vi "Run all tests CLI.vi"   [LabVIEW 2021]
uses:
  <vilib>/addons/_JKI Toolkits/Caraya/classes/Test Report/Test Report.lvclass
  <vilib>/addons/_JKI Toolkits/Caraya/run-tests/Run Test (Scalar Path).vi
  <vilib>/addons/_JKI Toolkits/Caraya/classes/Test Suite/Test Suite.lvclass
  <vilib>/Wiresmith Technology/G CLI/CLI Class/CLI.lvclass
  <vilib>/addons/_JKI Toolkits/Caraya/classes/Test Result/Test Result.lvclass
  <vilib>/addons/_JKI Toolkits/Caraya/Caraya.lvlib
types:
  T1 = enum32{"Invalid", "Standard", "Closed", "Hidden", "Minimized", "Maximized"}
  T2 = typedef "Caraya.lvlib/Test Result.lvclass/Node Results (Extended).ctl" = cluster{"Test Node":T3, "Assertions":T5[]}
  T3 = typedef "Caraya.lvlib/Test Result.lvclass/Test Node (Extended).ctl" = cluster{"Test Registration":T4, "Defined":bool, "Passed":bool, "properties":variant}
  T4 = typedef "Caraya.lvlib/Test Result.lvclass/Test Registration Data.ctl" = cluster{"Name":string, "Call Chain":string[], "Time Stamp":timestamp, "Test ID":string, "Caller ID":string}
  T5 = typedef "Caraya.lvlib/Test Result.lvclass/Assert Event Data (Extended).ctl" = cluster{"name":string, "passed":bool, "call-chain":string[], "test-error":errorcluster, "timestamp":timestamp, "assert-id":string, "test-id":string, "time":dbl, "message":string, "properties":variant, "measurements":variant, "user-defined":variant}
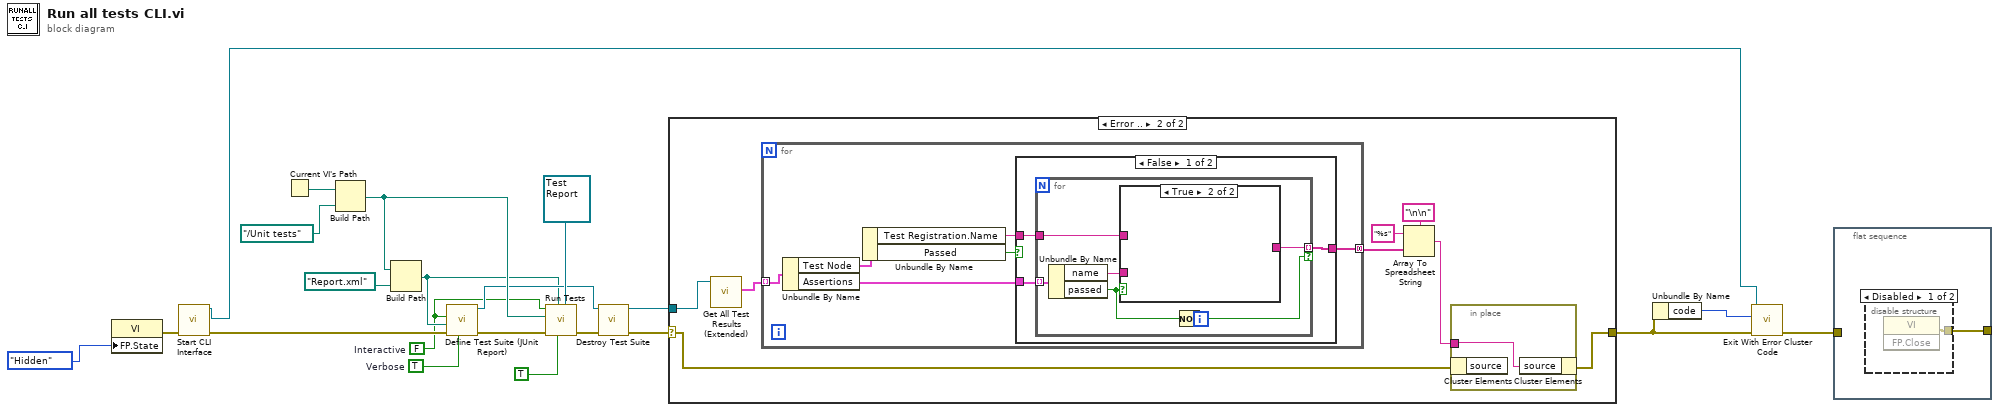
[diagram p0: block diagram]
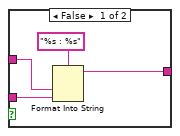
[diagram p3: hidden frame]
diagram:
  w12 = TRUE  # Verbose
  w1 = FALSE  # Interactive
  n1 = property class="VI"("FP.State"=T1."Hidden" ("Front Panel Window:State")) -> (error out=w8:errorcluster)  [unwired: 2 in, 1 out]
  n2 = call <vilib>:"Start CLI Interface.vi"("error in (no error)"=w8) -> ("error out"=w3:errorcluster, "CLI out"=w6:refnum<class "CLI.lvclass">)  [unwired: 7 in, 2 out]
  n3 = Current VI's Path() -> (path=w19:path)
  n4 = Build Path(base path=w19, name or relative path=path "../Unit tests") -> (appended path=w16:path)
  n5 = Build Path(base path=w16, name or relative path=path "Report.xml") -> (appended path=w11:path)
  n6 = call <vilib>:"Define Test Suite (JUnit Report).vi"("Verbose (F)"=w12, "error in (no error)"=w3, "Report Path"=w11, "Interactive"=w1) -> ("error out"=w10:errorcluster, "Test Suite"=w13:refnum<class "Test Suite.lvclass">)  [unwired: 5 in, 1 out]
  n7 = call-poly <vilib>:"Run Tests.vi"("Test Report"=refnum<class "Test Report.lvclass"> refnum, "Verbose"=TRUE, "Report Path"=w11, "error in"=w10, "Test Path"=w16, "Interactive (T)"=w1) -> ("error out"=w9:errorcluster)  [unwired: 4 in, 1 out]
  n8 = call-dynamic "Destroy Test Suite.vi"("error in (no error)"=w9, "Test Suite in"=w13) -> ("error out"=w5:errorcluster, "Test Suite Results"=w14:refnum<class "Test Result.lvclass">)  [unwired: 8 in]
  n9 = case shown="Error .." w5 {
    selector: w5 -> [w22 w25]
    tunnel: w14 -> [_ w30]
    tunnel: [w22 w23] -> w4
    frame No Error {
    }
    frame Error {
      n10 = call <vilib>:"Get All Test Results (Extended).vi"("Test Result in"=w30) -> ("Test Results"=w26:T2[])  [unwired: 8 in, 2 out]
      n11 = for {
        tunnel: w26 -> [w36] mode=indexing
        tunnel: [w32] -> w27 mode=concatenating
        n12 = Unbundle By Name(w36) -> ("Test Node"=w35:T3, "Assertions"=w37:T5[])
        n13 = Unbundle By Name(w35) -> ("Test Registration.Name"=w33:string, "Passed"=w34:bool)
        n14 = case shown="False" w34 {
          tunnel: w37 -> [w40 _]
          tunnel: w33 -> [w39 _]
          tunnel: [w38 _] -> w32
          frame False {
            n15 = for {
              tunnel: w40 -> [w46] mode=indexing
              tunnel: w39 -> [w44]
              tunnel: [w43] -> w38 mode=indexing if=w41
              n16 = Unbundle By Name(w46) -> ("name"=w45:string, "passed"=w42:bool)
              n17 = case shown="True" w42 {
                tunnel: w45 -> [w49 _]
                tunnel: w44 -> [w50 _]
                tunnel: [w47 _] -> w43
                frame False {
                  n18 = Format Into String(format string="%s : %s", w50, w49) -> (resulting string=w47:string)  [unwired: 2 in, 1 out]
                }
                frame True {
                }
              }
              n19 = Not(x=w42) -> (.not. x?=w41:bool)
            }
          }
          frame True {
          }
        }
      }
      n20 = Array To Spreadsheet String(delimiter (Tab)="\n\n", array=w27, 3:"%s" ("format string")) -> (spreadsheet string=w24:string)
      n21 = in-place {
        in-place-border: w24 -> [w31]
        n22 = in-place-cluster #1(w25) -> ()  [unwired: 1 out]
        n23 = in-place-cluster #1("source"=w31) -> (w23:errorcluster)
      }
    }
  }
  n24 = Unbundle By Name(w4) -> ("code"=w20:i32)
  n25 = call <vilib>:"Exit With Error Cluster Code.vi"("error in (no error)"=w4, "No Error Code (0)"=w20, "CLI in"=w6) -> ("error out"=w21:errorcluster)  [unwired: 8 in]
  n26 = flat-sequence {
    tunnel: [w51] -> _
    tunnel: w21 -> [_]
    frame #0 {
      n27 = disable-structure shown="Disabled" {
        disable-tunnel: [w52 _] -> w51
        frame Disabled {
          n28 = invoke class="VI" method="FP.Close"() -> (error out=w52:errorcluster)  [unwired: 3 in, 2 out]
        }
        frame Enabled {
        }
      }
    }
  }
